vi "plot generator main.vi"(11 "Shared Data from EMA":T2={"Impulse Positions"=[], "Parameter Impuls Series"=[], "Data File"={"Data Channels"=[], "Sample Rate"=0, "Channel List"=[]}, "desacc "={"Threshold 1 [Acc]"=7000.0, "Threshold 2 [% of TH1]"=60, "tolerance"=3, "Search WD "=0.1, " always use TH2"=FALSE, "Range"=2.0, "Max time"=120.0, "Min time"=20.0, "Velocity Threshold"=150}, "Experiment Parameters 2"={"Subject"="", "Strain"="", "Rotation plane"="", "Experimenter"="", "Trial"=0.0, "Time"=0.0}} {"Parameter Impuls Series"."Gain" format="%.1f"; "Parameter Impuls Series"."Offset" format="%.1f"}) -> (3 "Shared Data from EMA 2":T2={"Impulse Positions"=[], "Parameter Impuls Series"=[], "Data File"={"Data Channels"=[], "Sample Rate"=0, "Channel List"=[]}, "desacc "={"Threshold 1 [Acc]"=7000.0, "Threshold 2 [% of TH1]"=60, "tolerance"=3, "Search WD "=0.1, " always use TH2"=FALSE, "Range"=2.0, "Max time"=120.0, "Min time"=20.0, "Velocity Threshold"=150}, "Experiment Parameters 2"={"Subject"="", "Strain"="", "Rotation plane"="", "Experimenter"="", "Trial"=0.0, "Time"=0.0}} {"Parameter Impuls Series"."Gain" format="%.1f"; "Parameter Impuls Series"."Offset" format="%.1f"})   [LabVIEW 2013]
uses:
  Plugin Shared Data.ctl
  core/type-defs/TD_Impulse Parameter.ctl
  res/controls/impuls graph/impuls graph.xctl
  comm/impulse/impulse functions.lvlib
  core/core.lvlib
  plugin data.lvlib
panel:
  out "Impulse Plot 2":T1(xcontrol)
  out "Impulse Plot":T1(xcontrol)
  in  "Clear Button":bool
  in  "Add Button":bool
  in  "Parameter Impuls Series":T3=[{"Color"=4652800, "Visible"=TRUE, "Channel"=5, "Invert"=FALSE, "Desaccade"=FALSE, "Offset"=0.0, "Gain"=1.0}, {"Color"=16860, "Visible"=TRUE, "Channel"=13, "Invert"=FALSE, "Desaccade"=FALSE, "Offset"=0.0, "Gain"=1.0}, {"Color"=16711680, "Visible"=TRUE, "Channel"=21, "Invert"=FALSE, "Desaccade"=FALSE, "Offset"=0.0, "Gain"=1.0}] {"Gain" format="%.1f"; "Offset" format="%.1f"}
  in  "Impulse Direction":bool
  in  "Mean and STD":bool
  in  "Stop Button":bool
  # "Offset         Gain    Inv                    Channel                         Col   Vis   Sac"
  # "Pos"
  # "Neg"
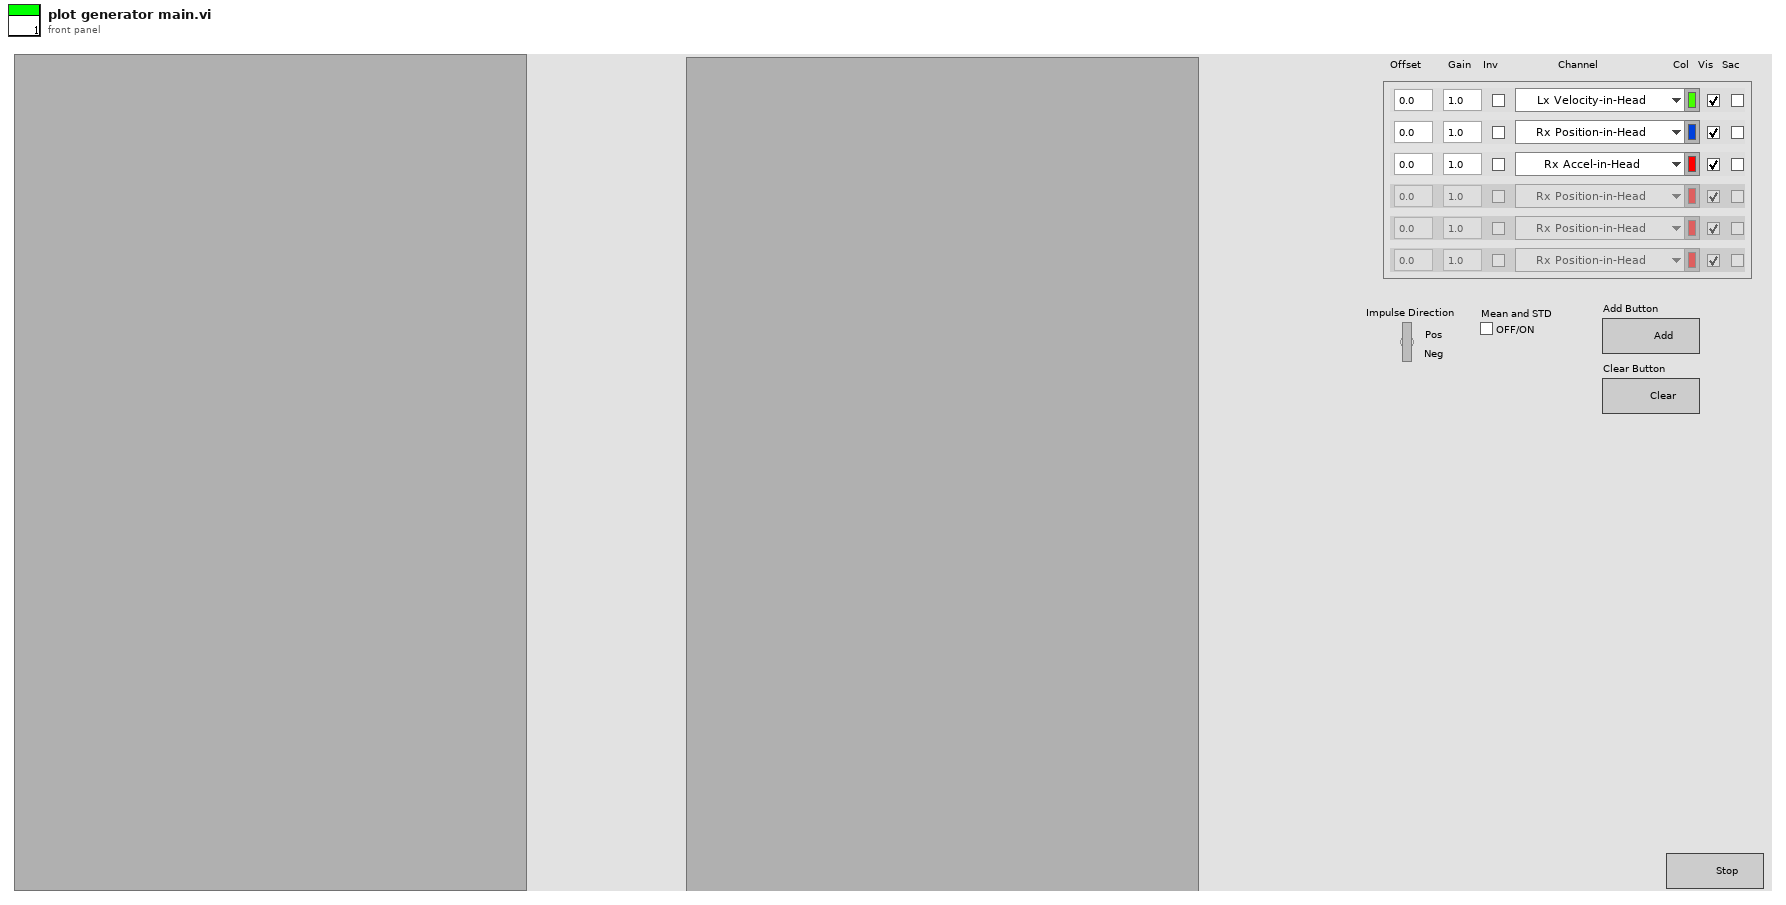
[diagram p1: front panel]
types:
  T1 = cluster{"Data":dbl[][], "Colour":u32, "Channel Name":string, "Sample Rate":dbl, "Visible":bool}[]
  T2 = typedef "plugin data.lvlib/Plugin Shared Data.ctl" = cluster{"Impulse Positions":cluster{"Start":i32, "End":i32, "Impulse Plane":enum16{"Other", "Yaw", "Pitch", "Roll", "LARP", "RALP"}, "Impulse Direction +ve?":bool, "Time offset":i32, "Amplitude offset":dbl}[], "Parameter Impuls Series":T3, "Data File":cluster{"Data Channels":dbl[][], "Sample Rate":i32, "Channel List":string[]}, "desacc ":cluster{"Threshold 1 [Acc]":dbl, "Threshold 2 [% of TH1]":i32, "tolerance":i32, "Search WD ":dbl, " always use TH2":bool, "Range":dbl, "Max time":dbl, "Min time":dbl, "Velocity Threshold":i32}, "Experiment Parameters 2":cluster{"Subject":string, "Strain":string, "Rotation plane":string, "Experimenter":string, "Trial":dbl, "Time":dbl}}
  T3 = typedef "core.lvlib/TD_Impulse Parameter.ctl" = cluster{"Color":u32, "Visible":bool, "Channel":u16, "Invert":bool, "Desaccade":bool, "Offset":dbl, "Gain":dbl}[]
  T4 = cluster{"Example Data":bool, "Temp":cluster{"Data":dbl[][], "Colour":u32, "Channel Name":string, "Sample Rate":dbl, "Visible":bool}[]}
  T5 = enum16{"Other", "Yaw", "Pitch", "Roll", "LARP", "RALP"}
  T6 = cluster{"Data Channels":dbl[][], "Sample Rate":i32, "Channel List":string[]}
  T7 = cluster{"Start":i32, "End":i32, "Impulse Plane":enum16{"Other", "Yaw", "Pitch", "Roll", "LARP", "RALP"}, "Impulse Direction +ve?":bool, "Time offset":i32, "Amplitude offset":dbl}[]
  T8 = cluster{"Threshold 1 [Acc]":dbl, "Threshold 2 [% of TH1]":i32, "tolerance":i32, "Search WD ":dbl, " always use TH2":bool, "Range":dbl, "Max time":dbl, "Min time":dbl, "Velocity Threshold":i32}
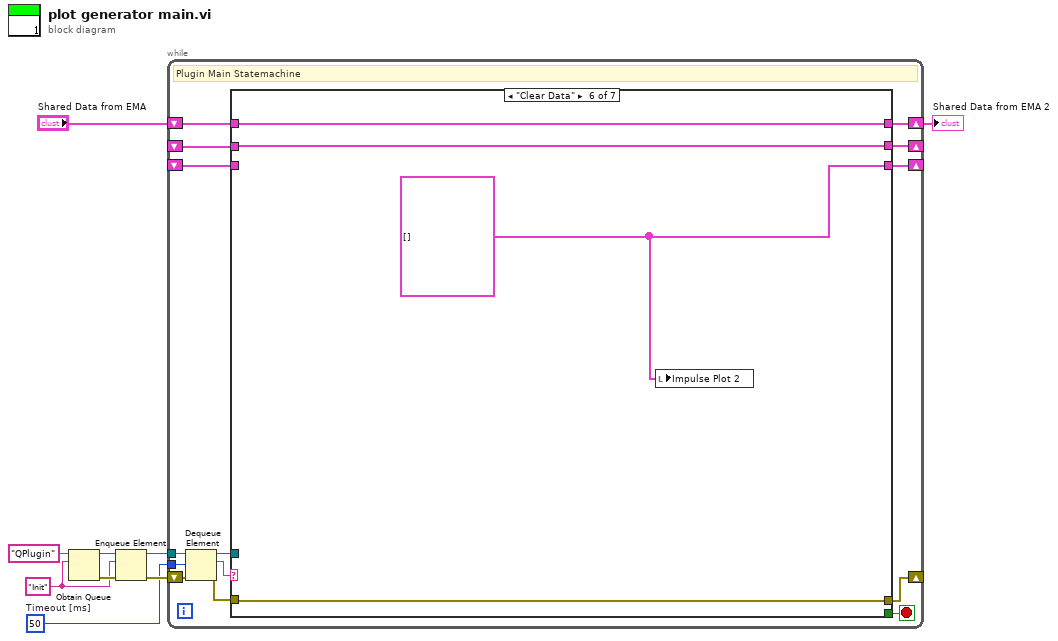
[diagram p0: block diagram]
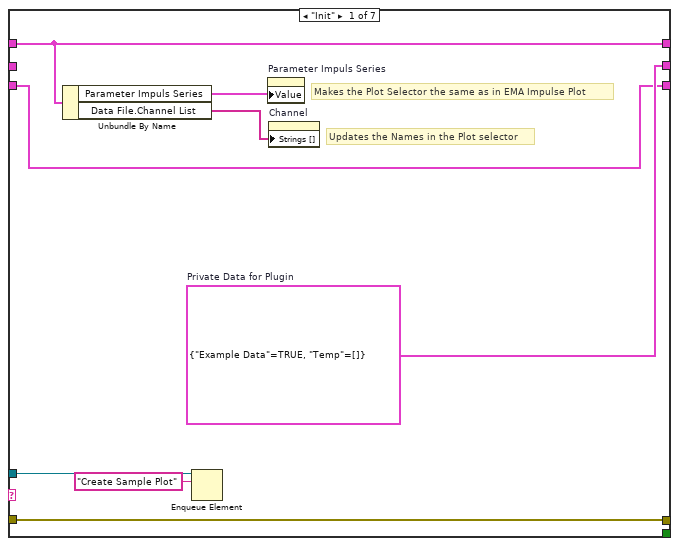
[diagram p2: hidden frame]
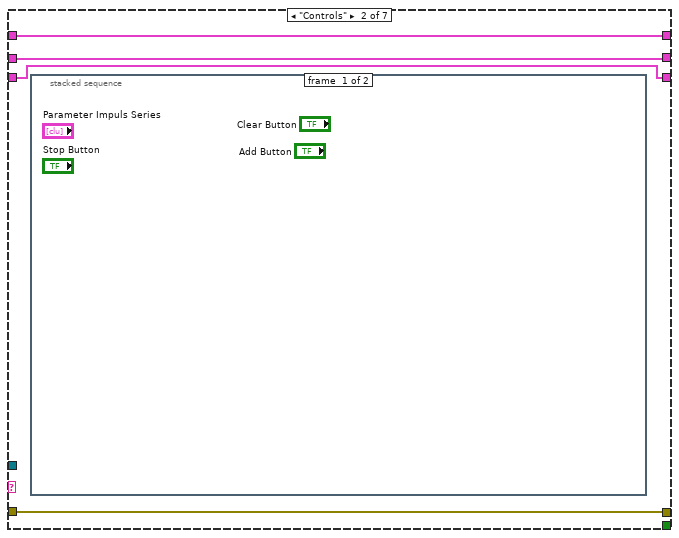
[diagram p3: hidden frame]
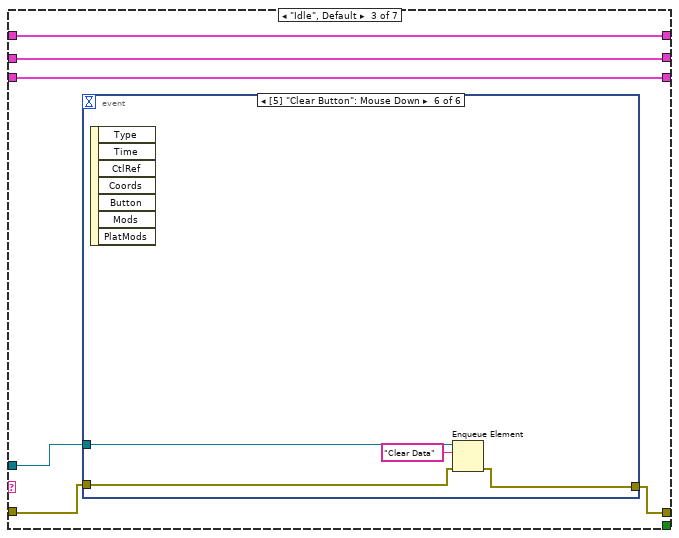
[diagram p5: hidden frame]
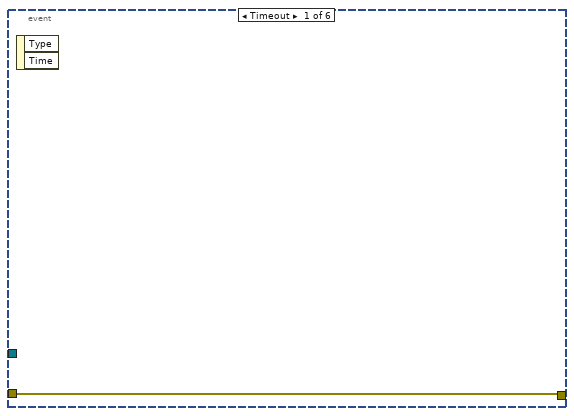
[diagram p6: hidden frame]
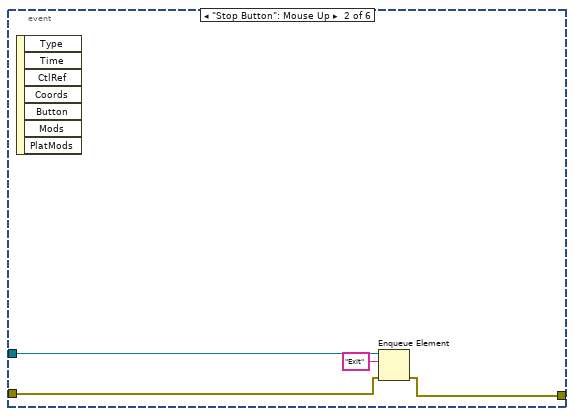
[diagram p7: hidden frame]
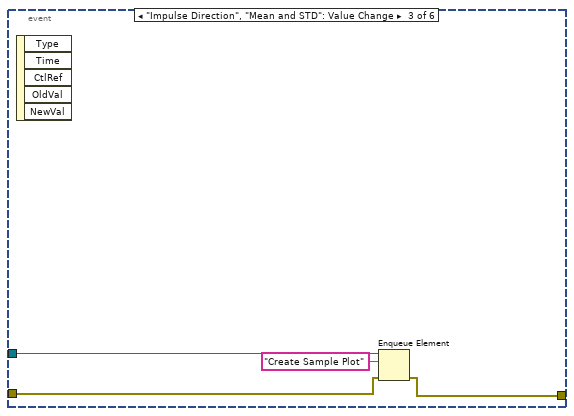
[diagram p8: hidden frame]
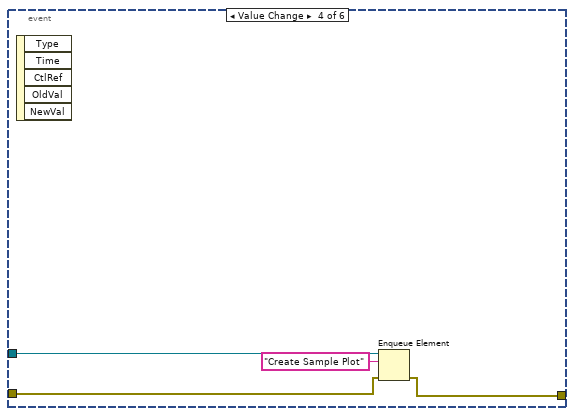
[diagram p9: hidden frame]
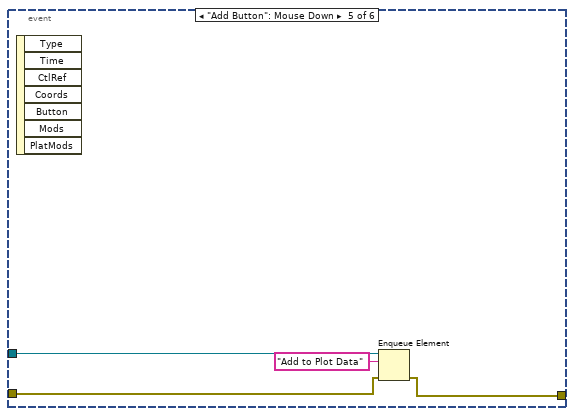
[diagram p10: hidden frame]
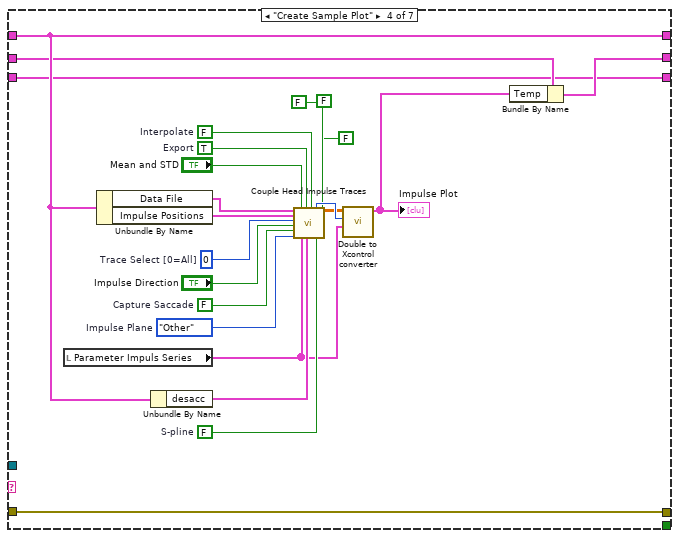
[diagram p11: hidden frame]
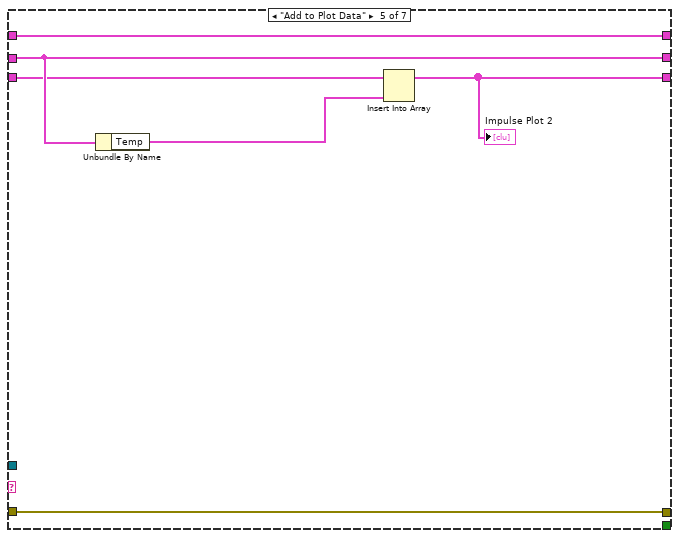
[diagram p12: hidden frame]
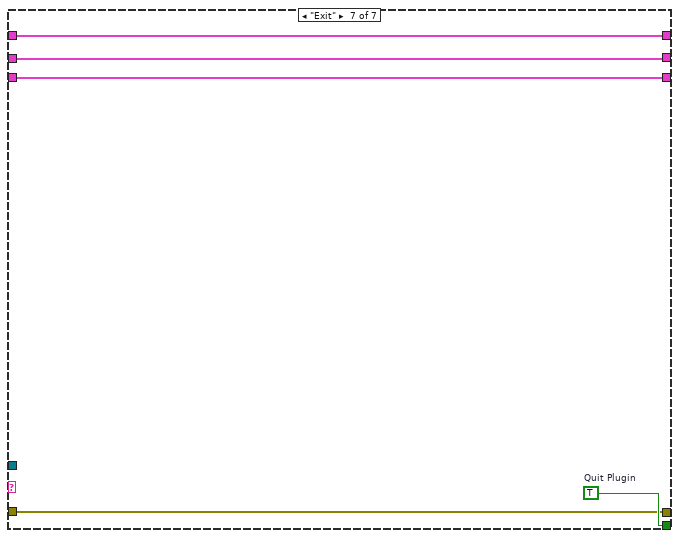
[diagram p13: hidden frame]
diagram:
  w3 = 50  # Timeout [ms]
  w7 = "Init"
  n1 = Obtain Queue(name (unnamed)="QPlugin", element data type=w7) -> (queue out=w8:refnum<queue>, error out=w9:errorcluster)  [unwired: 3 in, 1 out]
  n2 = Enqueue Element(queue=w8, element=w7, error in (no error)=w9) -> (queue out=w5:refnum<queue>, error out=w4:errorcluster)  [unwired: 1 in, 1 out]
  n3 = while {
    tunnel: w5 -> [w22]
    tunnel: w3 -> [w20]
    shift-right: [w16] -> _
    shift-left: w4 -> [w21]
    shift-right: [w15] -> _
    shift-left: _ -> [w14]
    shift-right: [w12] -> w1
    shift-left: "Shared Data from EMA" -> [w13]
    shift-right: [w11] -> _
    shift-left: _ -> [w10]
    stop <- w23 stop-if-true
    # "Plugin Main Statemachine"
    n4 = Dequeue Element(queue=w22, timeout in ms (-1)=w20, error in (no error)=w21) -> (queue out=w19:refnum<queue>, element=w18:string, error out=w17:errorcluster)  [unwired: 1 out]
    n5 = case shown="\"Clear Data\"" w18 {
      tunnel: [_ _ _ _ _ _ w100] -> w23
      tunnel: w19 -> [w29 _ w39 _ _ _ _]
      tunnel: w17 -> [w30 w33 w38 w85 w90 w93 w99]
      tunnel: [w30 w33 w37 w85 w90 w93 w99] -> w16
      tunnel: [w31 w34 w41 w68 w89 w94 w98] -> w15
      tunnel: w14 -> [_ w34 w41 w69 w89 w94 w98]
      tunnel: w13 -> [w27 w35 w40 w75 w91 w95 w97]
      tunnel: [w27 w35 w40 w75 w91 w95 w97] -> w12
      tunnel: [w24 w32 w36 w66 w86 w92 w96] -> w11
      tunnel: w10 -> [w24 w32 w36 w66 w88 _ w96]
      frame "Init" {
        w31 = T4 {"Example Data"=TRUE, "Temp"=[]}  # Private Data for Plugin
        # "Makes the Plot Selector the same as in EMA Impulse Plot"
        # "Updates the Names in the Plot selector"
        n6 = Unbundle By Name(w27) -> ("Parameter Impuls Series"=w26:T3, "Data File.Channel List"=w25:string[])
        n7 = Enqueue Element(queue=w29, element="Create Sample Plot") -> ()  [unwired: 2 in, 3 out]
        n8 = property on="Parameter Impuls Series" class="Arr (strict)"("Value"=w26) -> ()  [unwired: 2 in, 2 out]
        n9 = property on="Channel" class="Ring (strict)"("Strings []"=w25) -> ()  [unwired: 2 in, 2 out]
      }
      frame "Controls" {
        n10 = stacked-sequence {
          frame #0 {
          }
          frame #1 {
          }
        }
      }
      frame "Idle", Default {
        n11 = event shown="[5] \"Clear Button\": Mouse Down" {
          selector: _ -> [_ _ _ _ _ _]
          dyn-events: _ -> [_ _ _ _ _ _]
          timeout: _ -> [_ _ _ _ _ _]
          tunnel: w39 -> [_ w46 w50 w54 w58 w62]
          tunnel: w38 -> [w42 w44 w48 w52 w56 w60]
          tunnel: [w42 w43 w47 w51 w55 w59] -> w37
          event Timeout {
            n12 = event-data() -> ()  [unwired: 1 in, 2 out]
          }
          event "Stop Button": Mouse Up {
            n13 = event-data() -> ()  [unwired: 1 in, 7 out]
            n14 = Enqueue Element(queue=w46, element="Exit", error in (no error)=w44) -> (error out=w43:errorcluster)  [unwired: 1 in, 2 out]
          }
          event "Impulse Direction", "Mean and STD": Value Change {
            n15 = event-data() -> ()  [unwired: 1 in, 5 out]
            n16 = Enqueue Element(queue=w50, element="Create Sample Plot", error in (no error)=w48) -> (error out=w47:errorcluster)  [unwired: 1 in, 2 out]
          }
          event Value Change {
            n17 = event-data() -> ()  [unwired: 1 in, 5 out]
            n18 = Enqueue Element(queue=w54, element="Create Sample Plot", error in (no error)=w52) -> (error out=w51:errorcluster)  [unwired: 1 in, 2 out]
          }
          event "Add Button": Mouse Down {
            n19 = event-data() -> ()  [unwired: 1 in, 7 out]
            n20 = Enqueue Element(queue=w58, element="Add to Plot Data", error in (no error)=w56) -> (error out=w55:errorcluster)  [unwired: 1 in, 2 out]
          }
          event "Clear Button": Mouse Down {
            n21 = event-data() -> ()  [unwired: 1 in, 7 out]
            n22 = Enqueue Element(queue=w62, element="Clear Data", error in (no error)=w60) -> (error out=w59:errorcluster)  [unwired: 1 in, 2 out]
          }
        }
      }
      frame "Create Sample Plot" {
        w73 = FALSE  # S-pline
        w76 = FALSE  # Interpolate
        w77 = TRUE  # Export
        w79 = T5."Other"  # Impulse Plane
        w80 = FALSE  # Capture Saccade
        w82 = 0  # Trace Select [0=All]
        n23 = local read "Parameter Impuls Series"() -> (w71:T3)
        n24 = Unbundle By Name(w75) -> ("Data File"=w83:T6, "Impulse Positions"=w84:T7)
        n25 = Unbundle By Name(w75) -> ("desacc"=w74:T8)
        n26 = call "Couple Head Impulse Traces.vi"("Data Input"=w83, "Impulse Positions"=w84, "Trace Select"=w82, "Impulse Direction +ve?"="Impulse Direction", "Capture Saccade"=w80, "Impulse Plane"=w79, "Mean and STD"="Mean and STD", "Plot Selection 2"=w71, "Export"=w77, "desacc"=w74, "Interpolate"=w76, "S-pline"=w73, "desacc."=FALSE, "man. desacc.."=FALSE, "Display Saccade"=FALSE) -> ("No Impulses"=w72:i32, "Impulses"=w70:dbl[][])  [unwired: 1 in, 2 out]
        n27 = call "Double to Xcontrol converter.vi"("Parameter Impuls Series"=w71, "No Impulses"=w72, "Impulses"=w70) -> ("Array"=w67:T1)  [unwired: 8 in]
        "Impulse Plot" <- w67
        n28 = Bundle By Name(cluster=w69, "Temp"=w67) -> (w68:T4)
      }
      frame "Add to Plot Data" {
        n29 = Unbundle By Name(w89) -> ("Temp"=w87:T1)
        n30 = Insert Into Array(array=w88, new element=w87) -> (w86:T1)  [unwired: 1 in]
        "Impulse Plot 2" <- w86
      }
      frame "Clear Data" {
        w92 = T1 []
        n31 = local write "Impulse Plot 2"(w92) -> ()
      }
      frame "Exit" {
        w100 = TRUE  # Quit Plugin
      }
    }
  }
  "Shared Data from EMA 2" <- w1
